vi "WebView2 Demo Browser.vi"() -> ()   [LabVIEW 2024]
uses:
  <vilib>/sklein/WebView2/Webview2 Control/WebView2 Control.xctl
  <vilib>/sklein/WebView2/Webview2 Control/Paths.ctl
panel:
  out "Paths":T1
  in  "stop":bool
  in  "FWD":bool
  in  "Back":bool
  out "Status":string
  out "navigation complete":bool
  in  "Reload":bool
  in  "Go":bool
  in  "URL":string="http://ni.com"
  out "WebView2 Browser Control":string(xcontrol)
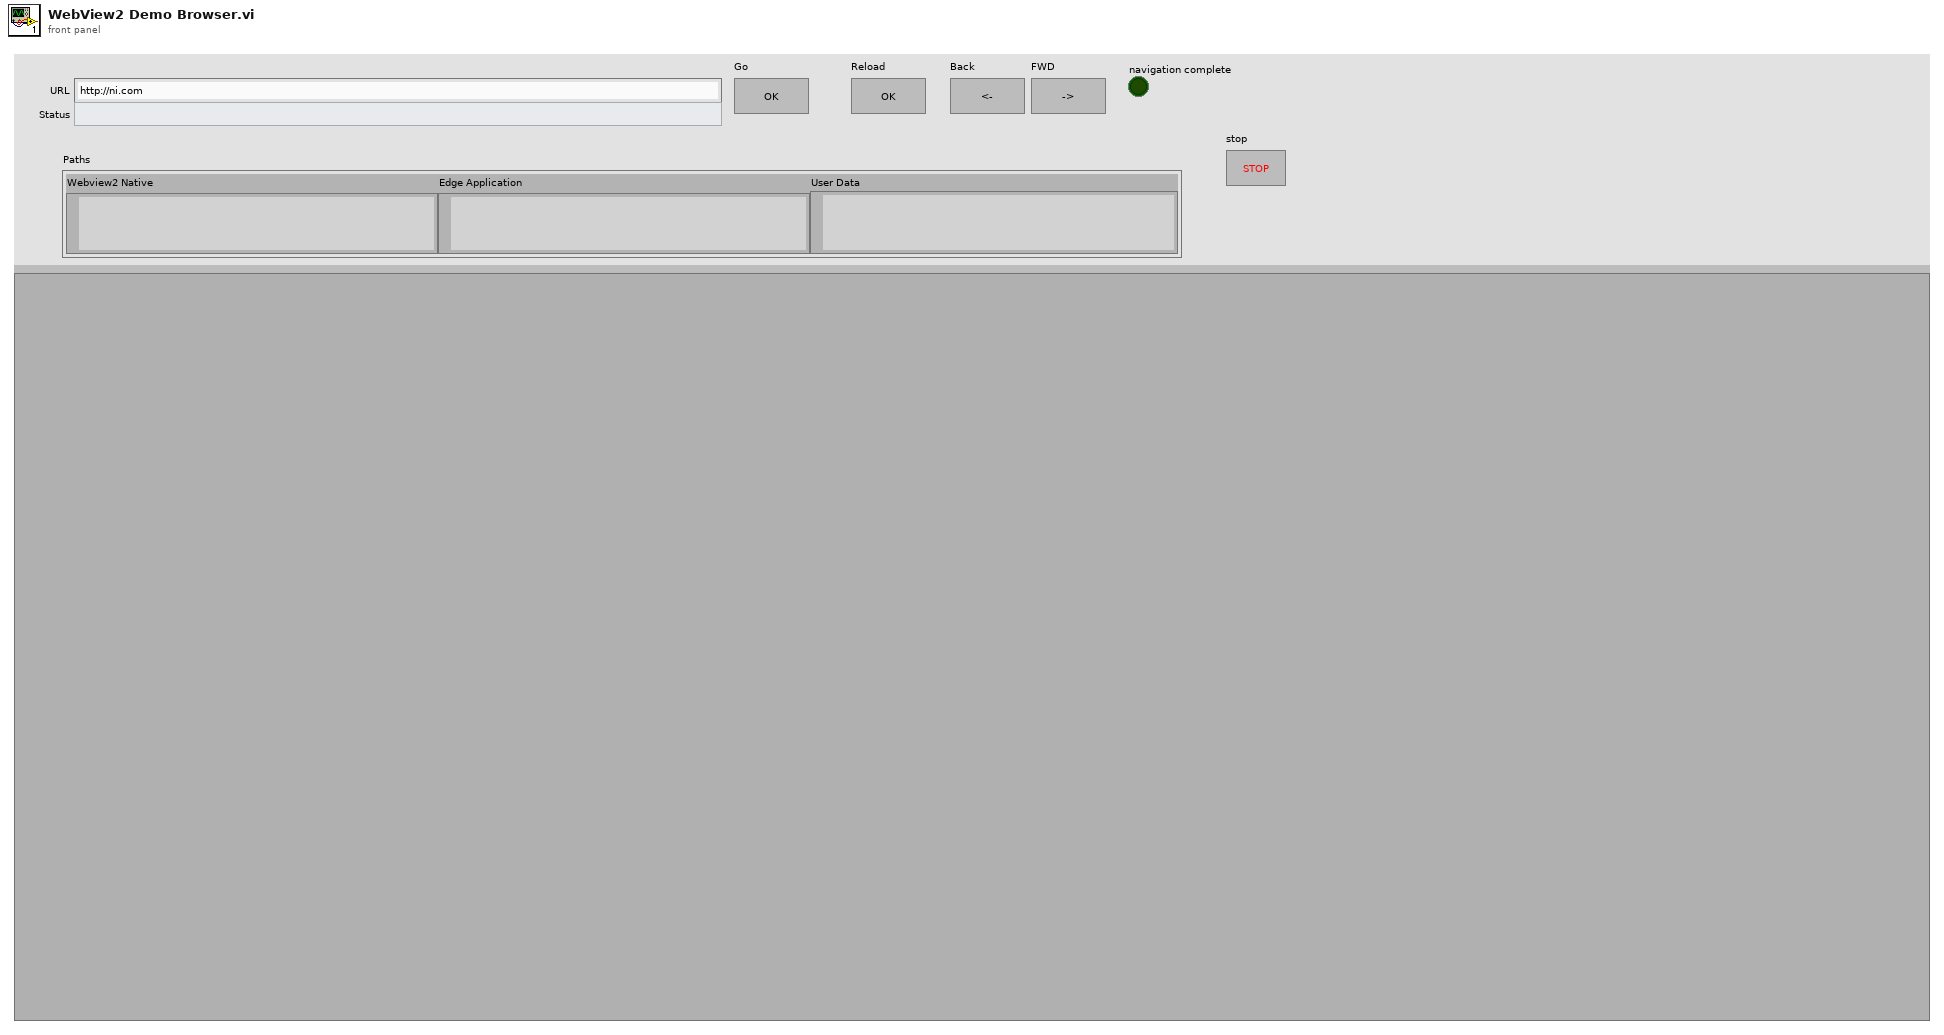
[diagram p1: front panel]
types:
  T1 = typedef "WebView2 Control.xctl/Paths.ctl" = cluster{"Webview2 Native":path, "Edge Application":path, "User Data":path}
  T2 = typedef "WebView2 Control.xctl/Events.ctl" = cluster{"Navigation Complete Event":refnum<user-event>, "Source Changed Event":refnum<user-event>, "Document Title Changed Event":refnum<user-event>, "Status Bar Text Changed":refnum<user-event>, "Web Message Received":refnum<user-event>, "Window Close Requested":refnum<user-event>, "DOM Loaded":refnum<user-event>, "Navigation Started Event":refnum<user-event>}
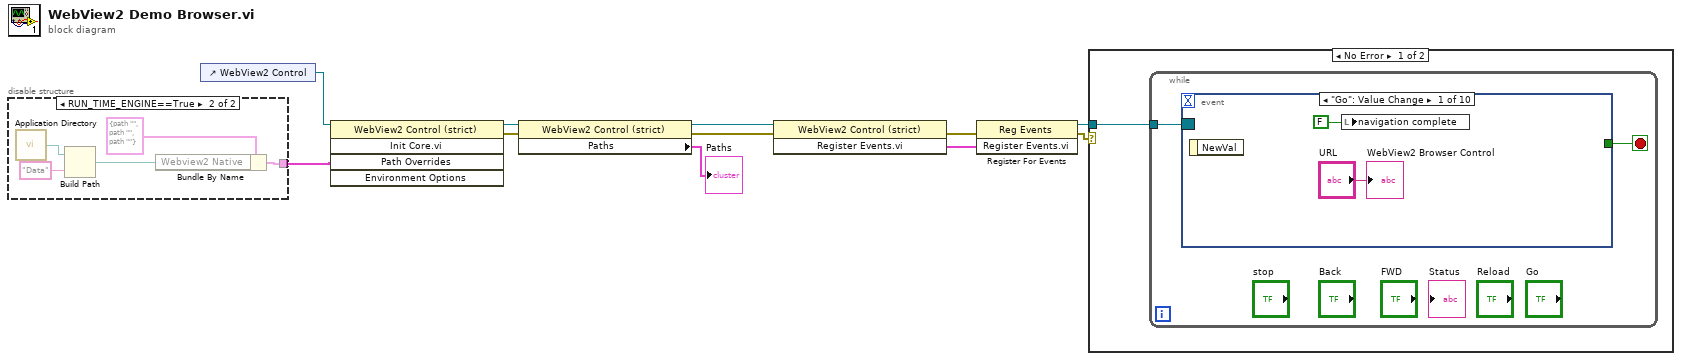
[diagram p0: block diagram]
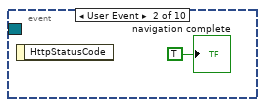
[diagram p3: hidden frame]
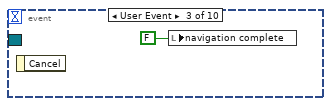
[diagram p4: hidden frame]
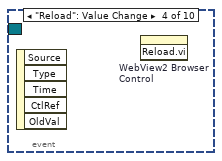
[diagram p5: hidden frame]
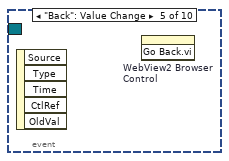
[diagram p6: hidden frame]
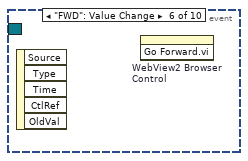
[diagram p7: hidden frame]
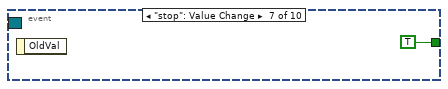
[diagram p8: hidden frame]
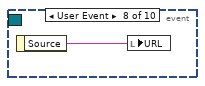
[diagram p9: hidden frame]
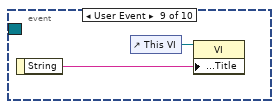
[diagram p10: hidden frame]
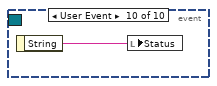
[diagram p11: hidden frame]
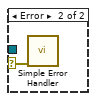
[diagram p12: hidden frame]
diagram:
  n1 = disable-structure shown="RUN_TIME_ENGINE==True" {
    disable-tunnel: [_ w15] -> w1
    frame condition #0 (active) {
    }
    frame condition #1 {
      n2 = call <vilib>:"Application Directory.vi"() -> ("Application Directory"=w13:path)
      n3 = Build Path(base path=w13, name or relative path="Data") -> (appended path=w14:path)
      n4 = Bundle By Name(cluster=T1 {"Webview2 Native"=path "", "Edge Application"=path "", "User Data"=path ""} ("Path Overrides"), "Webview2 Native"=w14) -> (w15:T1)
    }
  }
  n5 = control-ref of="WebView2 Control"() -> (w4:refnum<vi>)
  n6 = invoke class="WebView2 Control (strict)" method="Init Core.vi"(reference=w4, "Path Overrides"=w1) -> (reference out=w3:refnum<vi>, error out=w2:errorcluster)  [unwired: 3 in, 3 out]
  n7 = property class="WebView2 Control (strict)"(reference=w3, error in=w2) -> (reference out=w9:refnum<vi>, error out=w8:errorcluster, "Paths"=→"Paths":T1)
  n8 = invoke class="WebView2 Control (strict)" method="Register Events.vi"(reference=w9, error in=w8) -> (error out=w6:errorcluster, "Register Events.vi"=w5:T2)  [unwired: 1 in, 1 out]
  n9 = register-events(error in=w6, w5) -> (reference out=w11:refnum<event-registration>, error out=w10:errorcluster)  [unwired: 1 in]
  n10 = case shown="No Error" w10 {
    selector: w10 -> [_ w29]
    tunnel: w11 -> [w17 _]
    frame No Error {
      n11 = while {
        tunnel: w17 -> [w19]
        stop <- w18 stop-if-true
        n12 = event shown="[0] \"Go\": Value Change" {
          selector: w19 -> [_ _ _ _ _ _ _ _ _ _]
          dyn-events: _ -> [_ _ _ _ _ _ _ _ _ _]
          timeout: _ -> [_ _ _ _ _ _ _ _ _ _]
          tunnel: [_ _ _ _ _ _ TRUE _ _ _] -> w18
          event "Go": Value Change {
            n13 = event-data() -> ()  [unwired: 1 in, 1 out]
            n14 = local write "navigation complete"(FALSE ("navigation complete")) -> ()
            "WebView2 Browser Control" <- "URL"
          }
          event User Event {
            n15 = event-data() -> ()  [unwired: 1 in, 1 out]
            "navigation complete" <- TRUE ("navigation complete")
          }
          event User Event {
            n16 = event-data() -> ()  [unwired: 1 in, 1 out]
            n17 = local write "navigation complete"(FALSE ("navigation complete")) -> ()
          }
          event "Reload": Value Change {
            n18 = event-data() -> ()  [unwired: 1 in, 5 out]
            n19 = invoke on="WebView2 Browser Control" class="WebView2 Browser Control (stric" method="Reload.vi"() -> ()  [unwired: 3 in, 3 out]
          }
          event "Back": Value Change {
            n20 = event-data() -> ()  [unwired: 1 in, 5 out]
            n21 = invoke on="WebView2 Browser Control" class="WebView2 Browser Control (stric" method="Go Back.vi"() -> ()  [unwired: 3 in, 3 out]
          }
          event "FWD": Value Change {
            n22 = event-data() -> ()  [unwired: 1 in, 5 out]
            n23 = invoke on="WebView2 Browser Control" class="WebView2 Browser Control (stric" method="Go Forward.vi"() -> ()  [unwired: 3 in, 3 out]
          }
          event "stop": Value Change {
            n24 = event-data() -> ()  [unwired: 1 in, 1 out]
          }
          event User Event {
            n25 = event-data() -> ("Source"=w25:string)  [unwired: 1 in]
            n26 = local write "URL"(w25) -> ()
          }
          event User Event {
            n27 = event-data() -> ("String"=w26:string)  [unwired: 1 in]
            n28 = control-ref of="This VI"() -> (w27:refnum<vi>)
            n29 = property class="VI"(reference=w27, "Front Panel.Title"=w26) -> ()  [unwired: 1 in, 2 out]
          }
          event User Event {
            n30 = event-data() -> ("String"=w28:string)  [unwired: 1 in]
            n31 = local write "Status"(w28) -> ()
          }
        }
      }
    }
    frame Error {
      n32 = call <vilib>:"Simple Error Handler.vi"("error in (no error)"=w29) -> ()  [unwired: 4 in, 5 out]
    }
  }
